vi "Release.vi"(8 "error in (no error)":errorcluster, 11 "SECS Data Class in":refnum<class "SECS Data Class.lvclass">) -> (0 "error out":errorcluster)   [LabVIEW 2020, in "SECS Communication.lvlib" / "SECS Data Class.lvclass"]
uses:
  SECS Data Class.lvclass
  SECS Data Class.lvclass/SECS Data Class.ctl
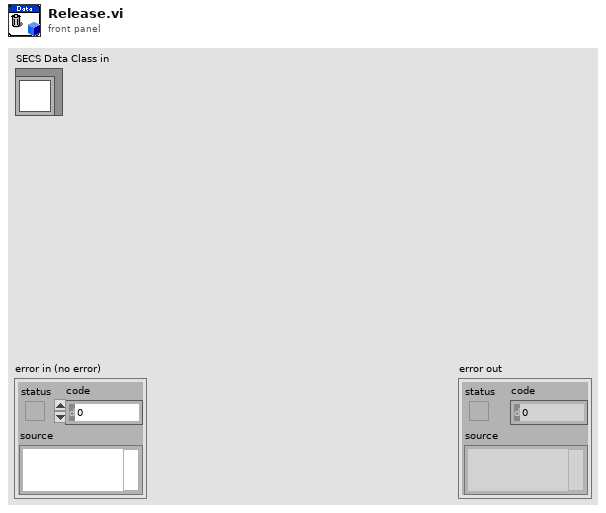
[diagram p1: front panel]
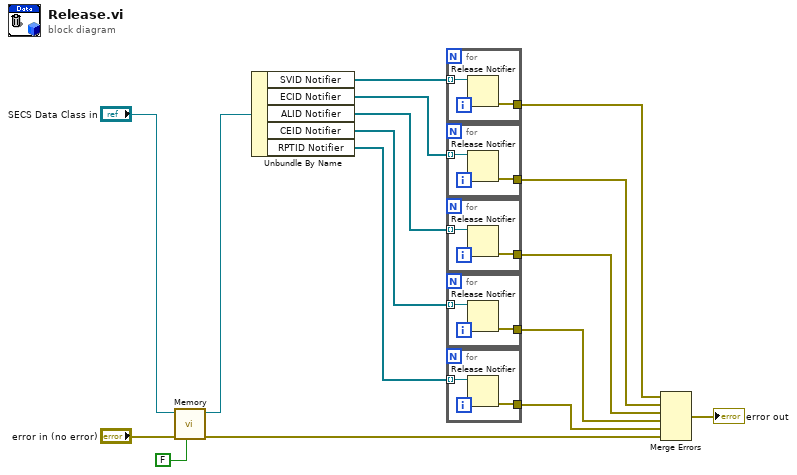
[diagram p0: block diagram]
diagram:
  n1 = call "Memory.vi"("Put"=FALSE, "error in (no error)"="error in (no error)", "SECS Data Class in"="SECS Data Class in") -> ("error out"=w2:errorcluster, "SECS Data Class out"=w3:refnum<class "SECS Data Class.lvclass">)  [unwired: 7 in]
  n2 = Unbundle By Name(w3) -> ("SVID Notifier"=w15:refnum<notifier>[], "ECID Notifier"=w14:refnum<notifier>[], "ALID Notifier"=w13:refnum<notifier>[], "CEID Notifier"=w9:refnum<notifier>[], "RPTID Notifier"=w7:refnum<notifier>[])
  n3 = for {
    tunnel: w15 -> [w18] mode=indexing
    tunnel: [w17] -> w10
    n4 = Release Notifier(notifier=w18) -> (error out=w17:errorcluster)  [unwired: 2 in, 2 out]
  }
  n5 = for {
    tunnel: w14 -> [w20] mode=indexing
    tunnel: [w19] -> w11
    n6 = Release Notifier(notifier=w20) -> (error out=w19:errorcluster)  [unwired: 2 in, 2 out]
  }
  n7 = for {
    tunnel: w13 -> [w21] mode=indexing
    tunnel: [w22] -> w12
    n8 = Release Notifier(notifier=w21) -> (error out=w22:errorcluster)  [unwired: 2 in, 2 out]
  }
  n9 = for {
    tunnel: w9 -> [w23] mode=indexing
    tunnel: [w24] -> w8
    n10 = Release Notifier(notifier=w23) -> (error out=w24:errorcluster)  [unwired: 2 in, 2 out]
  }
  n11 = for {
    tunnel: w7 -> [w25] mode=indexing
    tunnel: [w26] -> w6
    n12 = Release Notifier(notifier=w25) -> (error out=w26:errorcluster)  [unwired: 2 in, 2 out]
  }
  n13 = Merge Errors(w10, w11, w12, w8, w6, w2) -> (→"error out":errorcluster)
